vi "Send Voltage.vi"(8 "error in":errorcluster, 11 "69X_79X in":refnum<class "79XRP.lvclass">) -> (0 "error out":errorcluster, 3 "69X_79X out":refnum<class "79XRP.lvclass">)   [LabVIEW 2019, in "79XRP.lvlib" / "79XRP.lvclass"]
uses:
  Library/79XRP.lvclass
  C:/Users/Public/Documents/Development/builds/Instruments/PowerSupply.lvlibp/Library/PowerSupply.lvclass
  Accessors/Read Local Resource.vi
  Accessors/Write Local Resource.vi
  builds/Engine/Engine.lvlibp/Project/Engine.lvclass
  C:/Users/Public/Documents/Development/builds/Engine/Engine.lvlibp/Project/Engine.lvclass
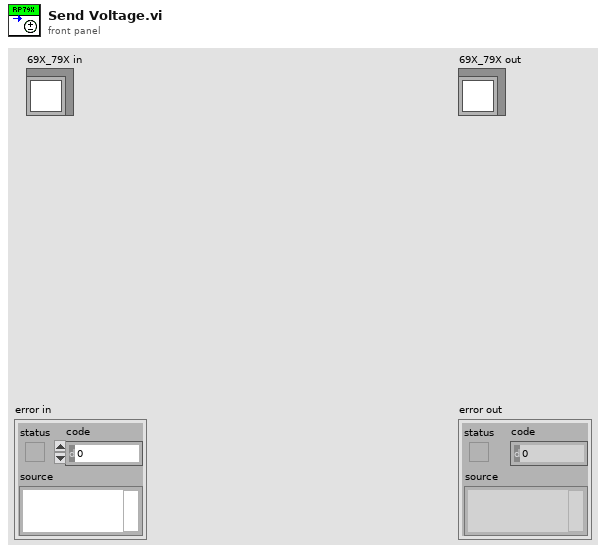
[diagram p1: front panel]
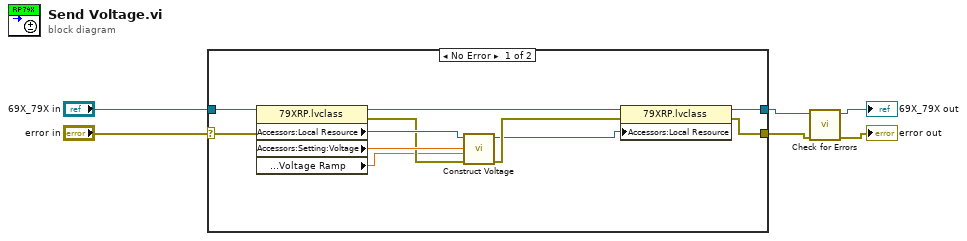
[diagram p0: block diagram]
diagram:
  n1 = case shown="No Error" "error in" {
    selector: "error in" -> [w16 w19]
    tunnel: "69X_79X in" -> [w17 w18]
    tunnel: [w13 w19] -> w2
    tunnel: [w14 w18] -> w1
    frame No Error {
      n2 = property class="79XRP.lvclass"(reference=w17, error in=w16) -> (reference out=w15:refnum<class "79XRP.lvclass">, error out=w10:errorcluster, "Accessors:Local Resource"=w12:refnum<visa-resource-name>, "Accessors:Setting:Voltage"=w11:dbl, "Accessors:Setting:Ramp:Voltage Ramp"=w7:dbl)
      n3 = call "Construct Voltage.vi"("error in (no error)"=w10, "Slew"=w7, "Voltage"=w11, "VISA resource name"=w12) -> ("error out"=w9:errorcluster, "VISA resource name out"=w8:refnum<visa-resource-name>)  [unwired: 6 in]
      n4 = property class="79XRP.lvclass"(reference=w15, error in=w9, "Accessors:Local Resource"=w8) -> (reference out=w14:refnum<class "79XRP.lvclass">, error out=w13:errorcluster)
    }
    frame Error {
    }
  }
  n5 = call "Check for Errors.vi"("error in"=w2, "Engine in"=w1) -> ("error out"=→"error out":errorcluster, "Engine out"=→"69X_79X out":refnum<class "79XRP.lvclass">)  [unwired: 8 in]
